vi "Read Move Speed.vi"(8 "error in (no error)":errorcluster, 11 "CAD Dispense in":refnum<class "CAD Dispense.lvclass">) -> (0 "error out":errorcluster, 2 "Move Speed":i32=30, 3 "CAD Dispense out":refnum<class "CAD Dispense.lvclass">)   [LabVIEW 2019, in "CAD Dispense.lvclass"]
uses:
  CAD Dispense.lvclass
  CAD Dispense.lvclass/CAD Dispense.ctl
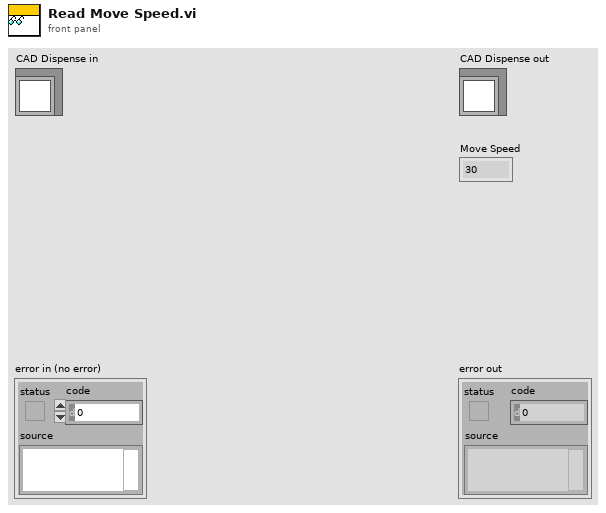
[diagram p1: front panel]
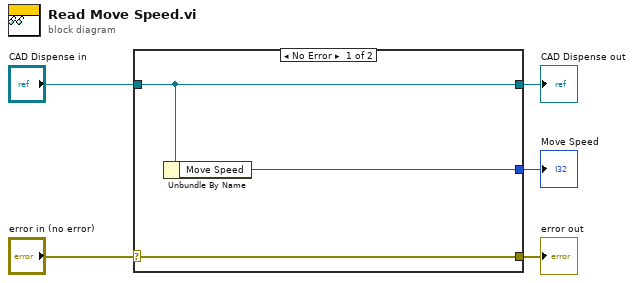
[diagram p0: block diagram]
diagram:
  n1 = case shown="No Error" "error in (no error)" {
    selector: "error in (no error)" -> [w8 w9]
    tunnel: [w8 w9] -> w4
    tunnel: [w7 w10] -> w2
    tunnel: "CAD Dispense in" -> [w7 w10]
    tunnel: [w6 _] -> w1
    frame No Error {
      n2 = Unbundle By Name(w7) -> ("Move Speed"=w6:i32)
    }
    frame Error {
    }
  }
  "error out" <- w4
  "CAD Dispense out" <- w2
  "Move Speed" <- w1
